vi "ADO Connection List Columns.vi"(8 "error in (no error)":errorcluster caption="错误输入（无错误）", 9 "table":string, 11 "Database Connection 输入":refnum<class "Database Connection.lvclass"> caption="DNL_LabVIEW Object in") -> (0 "error out":errorcluster caption="错误输出", 1 "Column Info":T1(array[cluster]) {"Type" items=["adEmpty"=0, "adTinyInt"=16, "adSmallInt"=2, "adInteger"=3, "adBigInt"=20, "adUnsignedTinyInt"=17, "adUnsignedSmallInt"=18, "adUnsignedInt"=19, "adUnsignedBigInt"=21, "adSingle"=4, "adDouble"=5, "adCurrency"=6, "adDecimal"=14, "adNumeric"=131, "adBoolean"=11, "adError"=10, "adUserDefined"=132, "adVariant"=12, "adIDispatch"=9, "adIUnknown"=13, "adGUID"=72, "adDate"=7, "adDBDate"=133, "adDBTime"=134, "adDBTimeStamp"=135, "adBSTR"=8, "adChar"=129, "adVarChar"=200, "adLongVarChar"=201, "adWChar"=130, "adVarWChar"=202, "adLongVarWChar"=203, "adBinary"=128, "adVarBinary"=204, "adLongVarBinary"=205, "adChapter"=136, "adFileTime"=64, "adPropVariant"=138, "adVarNumeric"=139, "adArray"=8192]}, 3 "Database Connection 输出":refnum<class "Database Connection.lvclass"> caption="DNL_LabVIEW Object out")   [LabVIEW 2011, in "Database Connection.lvclass"]
uses:
  Database Connection.lvclass
  Recordset/Database Recordset.lvclass
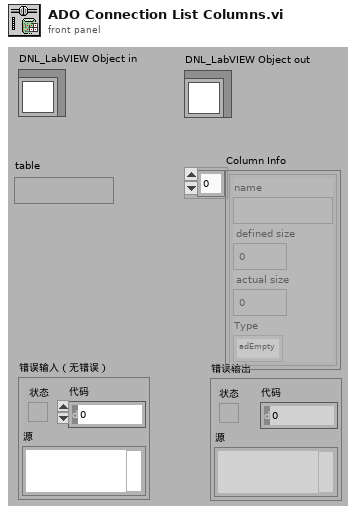
[diagram p1: front panel]
types:
  T1 = cluster{"name":string, "defined size":i32, "actual size":i32, "Type":i32}[]
  T2 = typedef "NI_Database_API.lvlib/DB Tools Cursor Type.ctl" = enum16{"forward-only", "keyset", "dynamic", "static"}
  T3 = cluster{"column count":i32, "record index":i32, "record count":i32, "bof?":bool, "eof?":bool, "cursor type":T2, "cache size":i32, "state":enum16{"closed", "open"}}
  T4 = cluster{"name":string, "defined size":i32, "actual size":i32, "Type":i32}
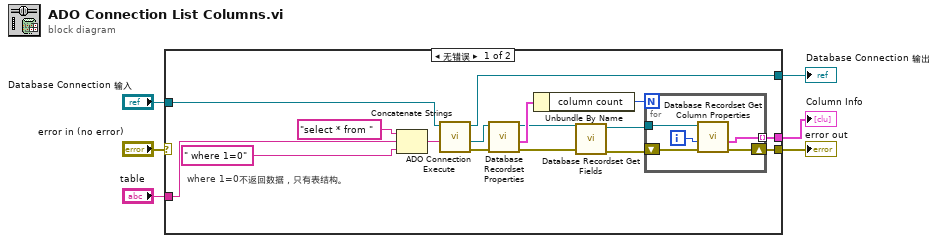
[diagram p0: block diagram]
diagram:
  n1 = case shown="无错误" "error in (no error)" {
    selector: "error in (no error)" -> [_ w29]
    tunnel: [w11 w29] -> w5
    tunnel: [w13 w28] -> w3
    tunnel: "Database Connection 输入" -> [w19 w28]
    tunnel: "table" -> [w20 _]
    tunnel: [w14 _] -> w1
    frame No Error {
      # "where 1=0不返回数据，只有表结构。"
      n2 = Concatenate Strings("select * from " ("Substring"), w20, " where 1=0" ("Substring")) -> (w18:string)
      n3 = call "ADO Connection Execute.vi"("CommandText"=w18, "Database Connection 输入"=w19) -> ("error out"=w17:errorcluster, "Database Recordset输出"=w16:refnum<class "Database Recordset.lvclass">, "Database Connection 输出"=w13:refnum<class "Database Connection.lvclass">)  [unwired: 7 in]
      n4 = call "Database Recordset Properties.vi"("error in (no error)"=w17, "Database Recordset 输入"=w16) -> ("error out"=w10:errorcluster, "recordset properties"=w15:T3, "Database Recordset 输出"=w9:refnum<class "Database Recordset.lvclass">)  [unwired: 7 in]
      n5 = Unbundle By Name(w15) -> ("column count"=w12:i32)
      n6 = call "Database Recordset Get Fields.vi"("error in (no error)"=w10, "Database Recordset 输入"=w9) -> ("error out"=w7:errorcluster, "Database Recordset 输出"=w8:refnum<class "Database Recordset.lvclass">)  [unwired: 8 in]
      n7 = for {
        N: w12 -> [_]
        tunnel: w8 -> [w27]
        tunnel: [w24] -> w14 mode=indexing
        shift-right: [w23] -> w11
        shift-left: w7 -> [w25]
        i -> [w26]
        n8 = call "Database Recordset Get Column Properties.vi"("error in (no error)"=w25, "Index"=w26, "Database Recordset 输入"=w27) -> ("error out"=w23:errorcluster, "column properties"=w24:T4)  [unwired: 6 in, 1 out]
      }
    }
    frame Error {
    }
  }
  "error out" <- w5
  "Database Connection 输出" <- w3
  "Column Info" <- w1
